vi "prime_lines_drug.vi"(8 "error in (no error)":errorcluster, 10 "GLOBAL SETTINGS IN":refnum<notifier>, 11 "EXP SETTINGS IN":refnum<notifier>) -> (0 "error out":errorcluster, 2 "GLOBAL SETTINGS OUT":refnum<notifier>, 3 "EXP SETTINGS OUT":refnum<notifier>)   [LabVIEW 2013]
uses:
  main_machine/type_defs/experiment_settings.ctl
  main_machine/type_defs/experiment_states.ctl
  main_machine/type_defs/global_settings.ctl
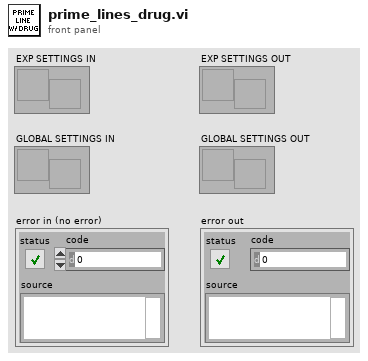
[diagram p1: front panel]
types:
  T1 = typedef "global_settings.ctl" = cluster{"# REACTORS":u32, "17X PORT":i32, "WASTE POSITION ":i32, "SECONDS BETWEEN SAMPLING":dbl, "FACS DIVA DIRECTORY":path, "DATA FILE":path, "REACTORS TO USE":u32[], "PULSE PERIOD":i32, "USE LIGHTS?":bool, "LED FILE":path, "LED CHANNELS":u32[], "PULSE LENGTH":i32, "SUMMARY FILE":path, "OUTGROWTH TIME POINTS":dbl, "SELECTION VALVE PORT":refnum<visa-resource-name>, "HTS PORT":refnum<visa-resource-name>, "DILUTION VOLUME (uL)":i32, "DILUTION FILE":path, "1X PORT":i32}
  T2 = typedef "experiment_settings.ctl" = cluster{"fcs file byte offset":i64, "LED Device Handle Out":u32, "START TIME":timestamp, "CURRENT VALVE":u32, "SAMPLE #":i32, "FCS FILE PATH":path, "TIME POINT":i32, "STATE":T3, "TIME TILL SAMPLE":dbl, "DILUTION  TABLE":dbl[][]}
  T3 = typedef "experiment_states.ctl" = enum16{"OUTGROWTH", "INDUCTION", "EXPERIMENT"}
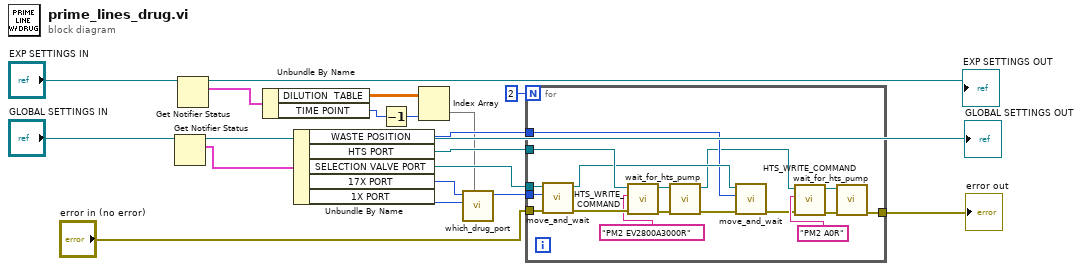
[diagram p0: block diagram]
diagram:
  n1 = Get Notifier Status(notifier="GLOBAL SETTINGS IN") -> (notifier out=→"GLOBAL SETTINGS OUT":refnum<notifier>, current notification=w8:T1)  [unwired: 1 in, 3 out]
  n2 = Get Notifier Status(notifier="EXP SETTINGS IN") -> (notifier out=→"EXP SETTINGS OUT":refnum<notifier>, current notification=w7:T2)  [unwired: 1 in, 3 out]
  n3 = Unbundle By Name(w7) -> ("DILUTION  TABLE"=w4:dbl[][], "TIME POINT"=w3:i32)
  n4 = Unbundle By Name(w8) -> ("WASTE POSITION"=w14:i32, "HTS PORT"=w13:refnum<visa-resource-name>, "SELECTION VALVE PORT"=w9:refnum<visa-resource-name>, "17X PORT"=w10:i32, "1X PORT"=w11:i32)
  n5 = Decrement(x=w3) -> (x-1=w2:i32)
  n6 = Index Array(array=w4, index (col)=w2) -> (element=w1:dbl[])  [unwired: 1 in]
  n7 = call "which_drug_port.vi"("DILUTION COLUMN"=w1, "1X PORT"=w11, "17X PORT"=w10) -> ("DRUG PORT"=w12:i32)  [unwired: 8 in]
  n8 = for {
    N: 2 -> [_]
    tunnel: w9 -> [w35]
    tunnel: w12 -> [w34]
    tunnel: w13 -> [w33]
    tunnel: w14 -> [w25]
    tunnel: [w21] -> w19
    tunnel: "error in (no error)" -> [w20]
    n9 = call "move_and_wait.vi"("Error IN"=w20, "MOVE TO POSITION"=w34, "VISA Resource IN"=w35) -> ("Error OUT"=w36:errorcluster, "Visa Resource OUT"=w27:refnum<visa-resource-name>)  [unwired: 6 in, 1 out]
    n10 = call "HTS_WRITE_COMMAND.vi"("Error IN"=w36, "Command"="PM2 EV2800A3000R", "HTS PORT IN"=w33) -> ("Error OUT"=w31:errorcluster, "HTS PORT OUT"=w30:refnum<visa-resource-name>)  [unwired: 6 in, 1 out]
    n11 = call "wait_for_hts_pump.vi"("error in (no error)"=w31, "HTS PORT IN"=w30) -> ("error out"=w26:errorcluster, "HTS PORT OUT"=w23:refnum<visa-resource-name>)  [unwired: 8 in]
    n12 = call "move_and_wait.vi"("Error IN"=w26, "MOVE TO POSITION"=w25, "VISA Resource IN"=w27) -> ("Error OUT"=w24:errorcluster)  [unwired: 6 in, 2 out]
    n13 = call "HTS_WRITE_COMMAND.vi"("Error IN"=w24, "Command"="PM2 A0R", "HTS PORT IN"=w23) -> ("Error OUT"=w29:errorcluster, "HTS PORT OUT"=w22:refnum<visa-resource-name>)  [unwired: 6 in, 1 out]
    n14 = call "wait_for_hts_pump.vi"("error in (no error)"=w29, "HTS PORT IN"=w22) -> ("error out"=w21:errorcluster)  [unwired: 8 in, 1 out]
  }
  "error out" <- w19
